vi "XW_Calib_Corr_TriMesh_PN.vi"(0 "B1 from Vel. Calib":dbl=1.36, 1 "A1 from Vel. Calib":dbl=2.21, 5 "n1 from Vel. Calib":dbl=0.42, 7 "A2 from Vel. Calib":dbl=2.25, 9 "B2 from Vel. Calib":dbl=1.4, 11 "n2 from Vel. Calib":dbl=0.41, 12 "Original triangles":T1[](array[typedef]), 13 "Zero angle dataset from map (used for calib. correction)":dbl[][](array[numeric])) -> (8 "Corrected triangles":T1[](array[typedef]), 10 "S*cos(q), S*sin(q), Tx, Ty":dbl[](array[numeric])=[1.0763223002323654, 0.0007524070719776288, -0.14779165640104555, -0.09827403757225917], 15 "Sx, Tx, Sy, Ty":dbl[](array[numeric])=[1.0000263372329348, -5.817138285027323e-05, 0.9999727510054321, 6.062261811624134e-05])   [LabVIEW 2010]
uses:
  Triangle2D.ctl
panel:
  # "This vi applies the matrix transformation to the ORIGINAL triangles in E1, E2 space and outputs the set of corrected triangles"
  # "Paul Nathan 17/02/10"
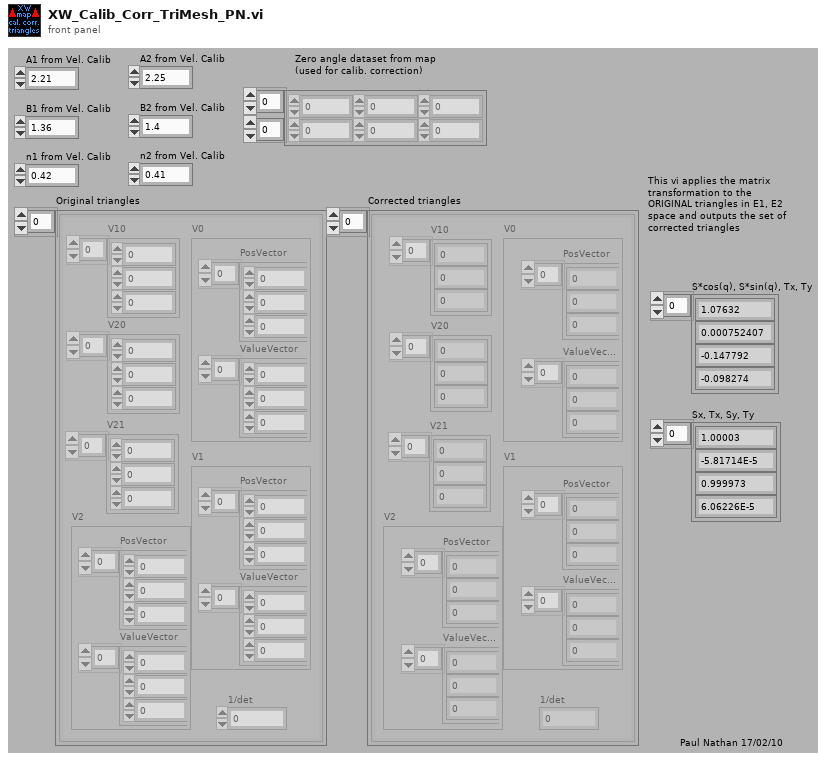
[diagram p1: front panel]
types:
  T1 = typedef "Triangle2D.ctl" = cluster{"V10":dbl[], "V20":dbl[], "1/det":dbl, "V0":cluster{"PosVector":dbl[], "ValueVector":dbl[]}, "V1":cluster{"PosVector":dbl[], "ValueVector":dbl[]}, "V2":cluster{"PosVector":dbl[], "ValueVector":dbl[]}, "V21":dbl[]}
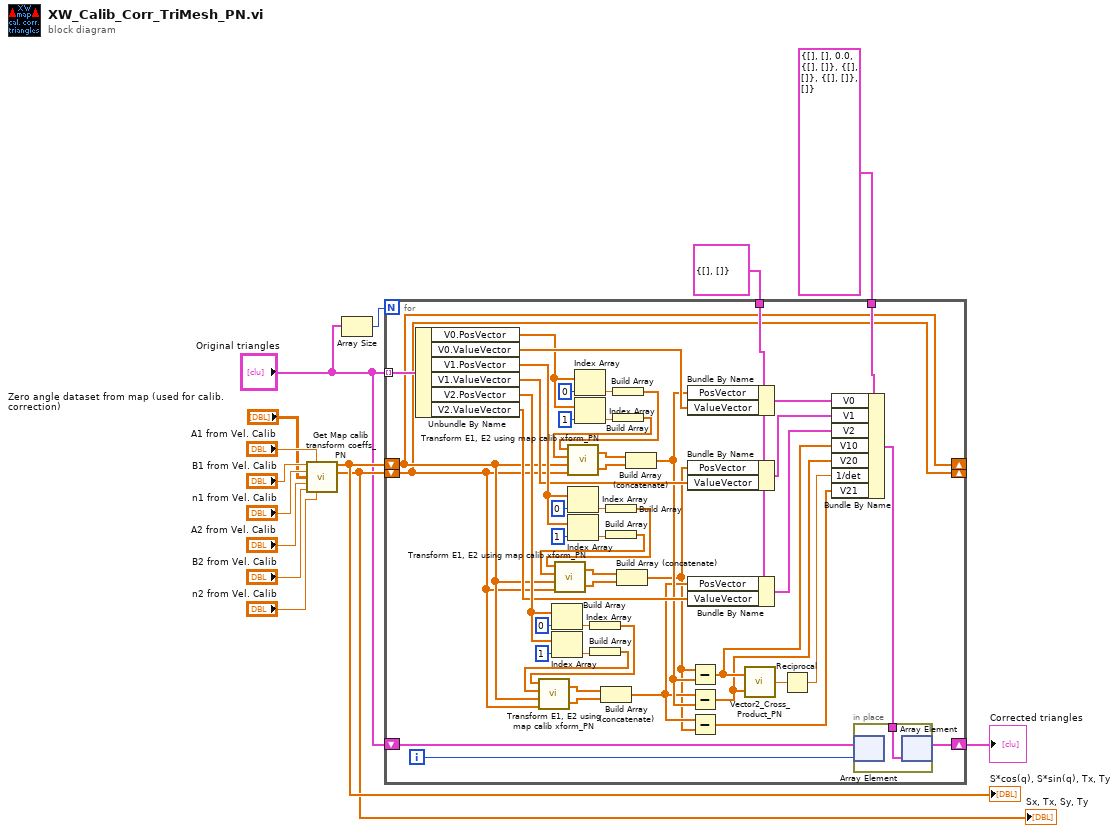
[diagram p0: block diagram]
diagram:
  n1 = call "Get Map calib transform coeffs_PN.vi"("B1 from Vel. Calib"="B1 from Vel. Calib", "A1 from Vel. Calib"="A1 from Vel. Calib", "n1 from Vel. Calib"="n1 from Vel. Calib", "Zero angle dataset from map (used for calib. correction)"="Zero angle dataset from map (used for calib. correction)", "A2 from Vel. Calib"="A2 from Vel. Calib", "B2 from Vel. Calib"="B2 from Vel. Calib", "n2 from Vel. Calib"="n2 from Vel. Calib") -> ("S*cos(q), S*sin(q), Tx, Ty"=w5:dbl[], "Sx, Tx, Sy, Ty"=w4:dbl[])  [unwired: 7 out]
  "S*cos(q), S*sin(q), Tx, Ty" <- w5
  "Sx, Tx, Sy, Ty" <- w4
  n2 = Array Size(array="Original triangles") -> (size(s)=w7:i32)
  n3 = for {
    N: w7 -> [_]
    tunnel: "Original triangles" -> [w64] mode=indexing
    shift-right: [w22] -> w2
    shift-left: "Original triangles" -> [w23]
    tunnel: cluster{"PosVector":dbl[], "ValueVector":dbl[]} {"PosVector"=[], "ValueVector"=[]} ("Vertex2D") -> [w51]
    tunnel: T1 {"V10"=[], "V20"=[], "1/det"=0.0, "V0"={"PosVector"=[], "ValueVector"=[]}, "V1"={"PosVector"=[], "ValueVector"=[]}, "V2"={"PosVector"=[], "ValueVector"=[]}, "V21"=[]} ("Triangle2D") -> [w53]
    shift-right: [w15] -> _
    shift-left: w4 -> [w15]
    shift-right: [w16] -> _
    shift-left: w5 -> [w16]
    i -> [w25]
    n4 = Unbundle By Name(w64) -> ("V0.PosVector"=w60:dbl[], "V0.ValueVector"=w63:dbl[], "V1.PosVector"=w42:dbl[], "V1.ValueVector"=w41:dbl[], "V2.PosVector"=w30:dbl[], "V2.ValueVector"=w29:dbl[])
    n5 = Index Array(array=w30, index=0) -> (element=w34:dbl)
    n6 = Index Array(array=w30, index=1) -> (element=w32:dbl)
    n7 = Index Array(array=w42, index=0) -> (element=w47:dbl)
    n8 = Index Array(array=w42, index=1) -> (element=w49:dbl)
    n9 = Index Array(array=w60, index=0) -> (element=w57:dbl)
    n10 = Index Array(array=w60, index=1) -> (element=w55:dbl)
    n11 = Build Array(w34) -> (w33:dbl[])
    n12 = Build Array(w32) -> (w31:dbl[])
    n13 = call "Transform E1, E2 using map calib xform_PN.vi"("Sx, Tx, Sy, Ty"=w15, "S*cos(q), S*sin(q), Tx, Ty"=w16, "E2/G2 + O2 orig"=w31, "E1/G1 + O1 orig"=w33) -> ("E2/G2 + O2 xformed"=w38:dbl[], "E1/G1 + O1 xformed"=w37:dbl[])
    n14 = Build Array (concatenate)(w37, w38) -> (w19:dbl[])
    n15 = Build Array(w47) -> (w48:dbl[])
    n16 = Build Array(w49) -> (w50:dbl[])
    n17 = call "Transform E1, E2 using map calib xform_PN.vi"("Sx, Tx, Sy, Ty"=w15, "S*cos(q), S*sin(q), Tx, Ty"=w16, "E2/G2 + O2 orig"=w50, "E1/G1 + O1 orig"=w48) -> ("E2/G2 + O2 xformed"=w43:dbl[], "E1/G1 + O1 xformed"=w44:dbl[])
    n18 = Build Array(w57) -> (w56:dbl[])
    n19 = Build Array(w55) -> (w54:dbl[])
    n20 = call "Transform E1, E2 using map calib xform_PN.vi"("Sx, Tx, Sy, Ty"=w15, "S*cos(q), S*sin(q), Tx, Ty"=w16, "E2/G2 + O2 orig"=w54, "E1/G1 + O1 orig"=w56) -> ("E2/G2 + O2 xformed"=w62:dbl[], "E1/G1 + O1 xformed"=w61:dbl[])
    n21 = Build Array (concatenate)(w44, w43) -> (w18:dbl[])
    n22 = Build Array (concatenate)(w61, w62) -> (w28:dbl[])
    n23 = Bundle By Name(cluster=w51, "PosVector"=w28, "ValueVector"=w63) -> (w52:cluster{"PosVector":dbl[], "ValueVector":dbl[]})
    n24 = Bundle By Name(cluster=w51, "PosVector"=w18, "ValueVector"=w41) -> (w40:cluster{"PosVector":dbl[], "ValueVector":dbl[]})
    n25 = Bundle By Name(cluster=w51, "PosVector"=w19, "ValueVector"=w29) -> (w39:cluster{"PosVector":dbl[], "ValueVector":dbl[]})
    n26 = Subtract(x=w18, y=w28) -> (x-y=w27:dbl[])
    n27 = Subtract(x=w19, y=w28) -> (x-y=w26:dbl[])
    n28 = Subtract(x=w19, y=w18) -> (x-y=w17:dbl[])
    n29 = call "Vector2_Cross_Product_PN.vi"("V (2D)"=w26, "U (2D)"=w27) -> ("U X V (2D)"=w21:dbl)
    n30 = Reciprocal(x=w21) -> (1/x=w20:dbl)
    n31 = Bundle By Name(cluster=w53, "V0"=w52, "V1"=w40, "V2"=w39, "V10"=w27, "V20"=w26, "1/det"=w20, "V21"=w17) -> (w24:T1)
    n32 = in-place {
      in-place-border: w24 -> [w65]
      n33 = in-place-array #1(w23, w25) -> ()  [unwired: 1 out]
      n34 = in-place-array #1(w65) -> (w22:T1[])  [unwired: 1 out]
    }
  }
  "Corrected triangles" <- w2
